vi "libssh2_knownhost_readfile.vi"(8 "error in (no error)":errorcluster, 9 "type (OpenSSH)":T1, 10 "filename":path, 11 "known hosts collection":T2) -> (0 "error out":errorcluster, 2 "hosts added":i32)   [LabVIEW 2013, in "libssh2.lvlib"]
doc: "Reads a collection of known hosts from the specified file and adds them to the collection of known hosts."
uses:
  libssh2.lvlib
  Known Host Collection Refnum.ctl
  Known Host File Type.ctl
  Global Settings.vi
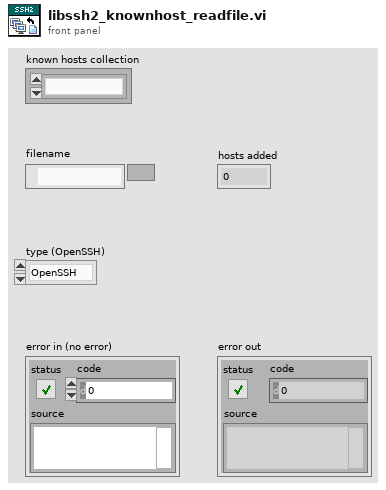
[diagram p1: front panel]
types:
  T1 = typedef "libssh2.lvlib/Known Host File Type.ctl" = enum16{"OpenSSH"}
  T2 = typedef "libssh2.lvlib/Known Host Collection Refnum.ctl" = refnum<k1>
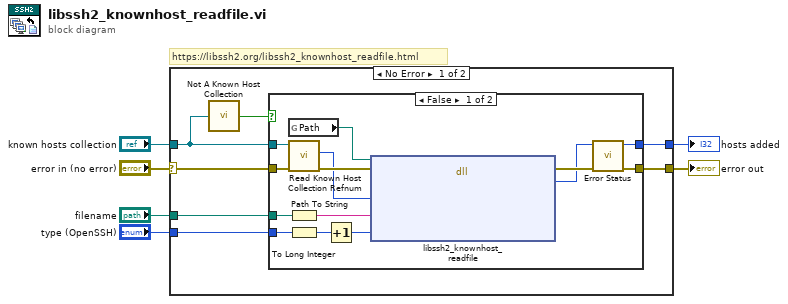
[diagram p0: block diagram]
diagram:
  # "https://libssh2.org/libssh2_knownhost_readfile.html"
  n1 = case shown="No Error" "error in (no error)" {
    selector: "error in (no error)" -> [w11 w29]
    tunnel: [w9 _] -> w6
    tunnel: [w10 w29] -> w5
    tunnel: "filename" -> [w13 _]
    tunnel: "type (OpenSSH)" -> [w12 _]
    tunnel: "known hosts collection" -> [w8 _]
    frame No Error {
      n2 = call "Not A Known Host Collection.vi"("known hosts collection"=w8) -> ("Not a Known Hosts Collection?"=w7:bool)
      n3 = case shown="False" w7 {
        tunnel: w13 -> [w26 _]
        tunnel: w12 -> [w25 _]
        tunnel: w8 -> [w23 _]
        tunnel: w11 -> [w21 w28]
        tunnel: [w19 w28] -> w10
        tunnel: [w17 _] -> w9
        frame False {
          n4 = global read "Global Settings.vi" "Path"() -> (w20:path)
          n5 = call "Read Known Host Collection Refnum.vi"("error in (no error)"=w21, "known hosts collection"=w23) -> ("error out"=w24:errorcluster, "LIBSSH2_KNOWNHOSTS*"=w22:u64)  [unwired: 8 in]
          n6 = Path To String(path=w26) -> (string=w16:string)
          n7 = To Long Integer(number=w25) -> (32bit integer=w14:i32)
          n8 = Increment(x=w14) -> (x+1=w15:i32)
          n9 = dll-call lib="C:/Users/pasca/source/repos/libssh2-labview/libssh2/libssh2**.*" fn="libssh2_knownhost_readfile"(path in=w20, error in=w24, "hosts"=w22, "filename"=w16, "type"=w15) -> (error out=w27:errorcluster, "return value"=w18:i32)  [unwired: 4 in, 1 out]
          n10 = call "Error Status.vi"("error in (no error)"=w27, "return value"=w18) -> ("error out"=w19:errorcluster, "return value out"=w17:i32)  [unwired: 8 in]
        }
        frame True {
        }
      }
    }
    frame Error {
    }
  }
  "hosts added" <- w6
  "error out" <- w5
